vi "Flatten Zip File to String.vi"(8 "error in":errorcluster, 10 "Path":path) -> (0 "error out":errorcluster, 2 "String":string)   [LabVIEW 2016, in "Server Controller.lvlib" / "Server Controller.lvclass"]
uses:
  Server Controller.lvclass
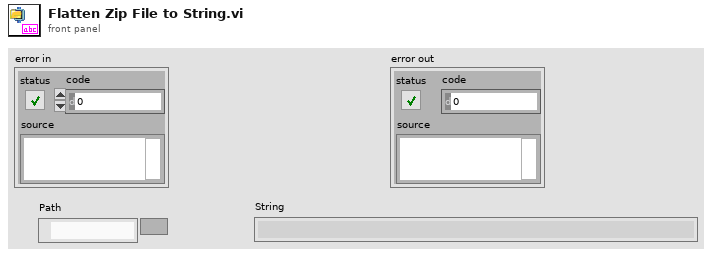
[diagram p1: front panel]
types:
  T1 = enum16{"open", "replace", "create", "open or create", "replace or create", "replace or create with confirmation"}
  T2 = enum16{"big-endian, network order", "native, host order", "little-endian"}
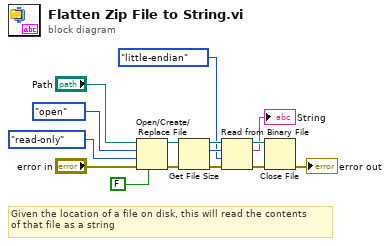
[diagram p0: block diagram]
diagram:
  # "Given the location of a file on disk, this will read the contents\nof that file as a string"
  n1 = Open/Create/Replace File(file path (use dialog)="Path", error in="error in", operation (0:open)=T1."open", access (0:read/write)=enum16{"read/write", "read-only", "write-only"}."read-only", disable buffering (F)=FALSE) -> (refnum out=w13:refnum<file>, error out=w3:errorcluster)  [unwired: 1 in, 1 out]
  n2 = Get File Size(file=w13, error in=w3) -> (refnum out=w12:refnum<file>, size (in bytes)=w11:i64, 0:w2:errorcluster)
  n3 = Read from Binary File(8:w2, 9:T2."little-endian" ("byte order (0:big-endian, network order)"), 10:w11, 11:w12) -> (0:w14:errorcluster, 2:→"String":string, 3:w15:refnum<file>)  [unwired: 2 in, 1 out]
  n4 = Close File(refnum=w15, error in=w14) -> (error out=→"error out":errorcluster)  [unwired: 1 out]
